vi "emi_Error finder Single.vi"(5 "Error Code":i32, 9 "error in (no error)":errorcluster) -> (6 "code":i32, 8 "In List":bool, 10 "error out":errorcluster, 13 "Is error":bool)   [LabVIEW 2010]
doc: "Find if error is one or severla error codes. Does not modify the error on the wire"
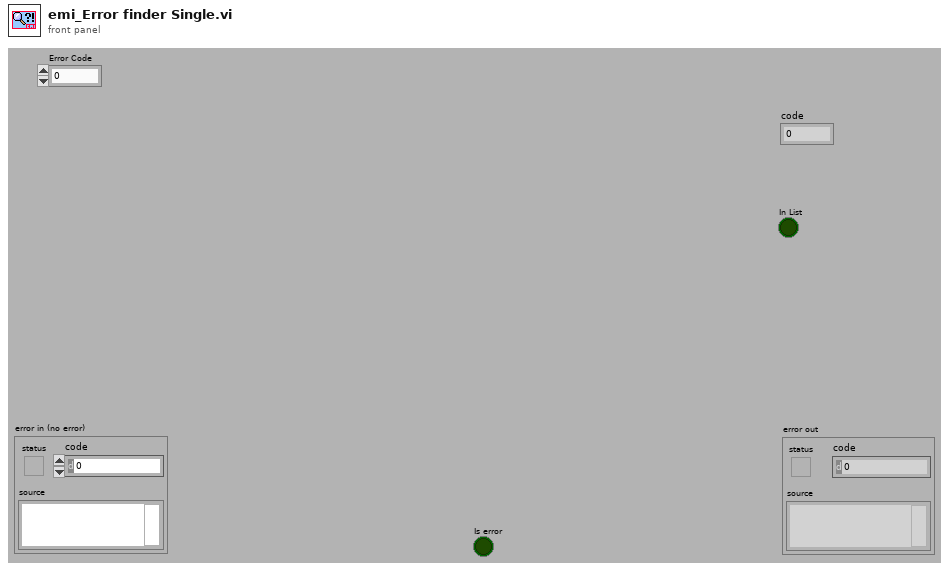
[diagram p1: front panel]
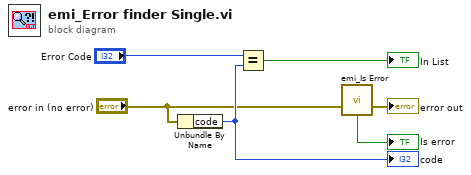
[diagram p0: block diagram]
diagram:
  n1 = Unbundle By Name("error in (no error)") -> ("code"=w6:i32)
  "code" <- w6
  n2 = Equal?(x="Error Code", y=w6) -> (x = y?=→"In List":bool)
  n3 = call "emi_Is Error.vi"("error in (no error)"="error in (no error)") -> ("error out"=→"error out":errorcluster, "Is Error"=→"Is error":bool)  [unwired: 13 in]
